vi "TR_KeyboardStatus.vi"(11 "Mouse in":refnum<class "Keyboard.lvclass">) -> ()   [LabVIEW 2021, in "InputDevice.lvlib" / "Keyboard.lvclass"]
uses:
  Keyboard.lvclass
  8ae88d8c-86e8-4183-9e02-5cb064982b42.vi
  <vilib>/Utility/inputDevices.llb/keyboardAcquire.vi
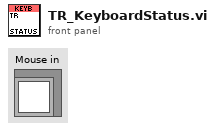
[diagram p1: front panel]
types:
  T1 = typedef "Keyboard.lvclass/data.ctl" = cluster{"DeviceID":refnum<k1>, "Key Pressed":refnum<user-event>, "KeyPressedEvents":refnum<event-registration>, "StopNotifier":refnum<notifier>}
  T2 = enum16{"0", "1", "2", "3", "4", "5", "6", "7", "8", "9", "A", "B", "C", "D", "E", "F", "G", "H", "I", "J", "K", "L", "M", "N", "O", "P", "Q", "R", "S", "T", "U", "V", "W", "X", "Y", "Z", "F1", "F2", "F3", "F4", "F5", "F6", "F7", "F8", "F9", "F10", "F11", "F12", "F13", "F14", "F15", "ADD", "BACK", "BACKSLASH", "CAPITAL", "COMMA", "DECIMAL", "DELETE", "DIVIDE", "DOWN", "END", "EQUALS", "ESCAPE", "GRAVE (`)", "HOME", "INSERT", "LBRACKET", "LCONTROL", "LEFT", "L ALT", "LSHIFT", "LWIN", "MINUS", "MULTIPLY", "NEXT", "NUMLOCK", "NUMPAD_0", "NUMPAD_1", "NUMPAD_2", "NUMPAD_3", "NUMPAD_4", "NUMPAD_5", "NUMPAD_6", "NUMPAD_7", "NUMPAD_8", "NUMPAD_9", "PAUSE", "PERIOD", "PRIOR (PG UP)", "RBRACKET", "RCONTROL", "RETURN", "RIGHT", "R ALT", "RSHIFT", "RWIN", "SCROLL", "SEMICOLON", "SLASH", "SPACE", "SUBTRACT", "TAB", "UP", "ENTER (num pad)", "' (quote)"}[]
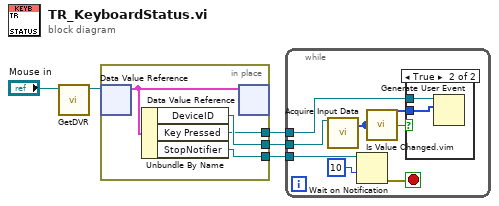
[diagram p0: block diagram]
diagram:
  n1 = call "GetDVR.vi"("Mouse"="Mouse in") -> ("DVR"=w4:refnum<data-value>)  [unwired: 9 in, 1 out]
  n2 = in-place {
    in-place-border: [w9] -> w3
    in-place-border: [w8] -> w2
    in-place-border: [w7] -> w1
    n3 = in-place-dvr #1(w4) -> (w6:T1)  [unwired: 1 out]
    n4 = Unbundle By Name(w6) -> ("DeviceID"=w9:refnum<k1>, "Key Pressed"=w8:refnum<user-event>, "StopNotifier"=w7:refnum<notifier>)
    n5 = in-place-dvr #1(w6) -> ()  [unwired: 2 out]
  }
  n6 = while {
    tunnel: w3 -> [w16]
    tunnel: w2 -> [w14]
    tunnel: w1 -> [w11]
    stop <- w12 stop-if-true
    n7 = call-poly <vilib>:"Acquire Input Data.vi"("device ID"=w16) -> ("keys pressed"=w13:T2)  [unwired: 16 in, 2 out]
    n8 = Wait on Notification(notifier=w11, timeout in ms (-1)=10) -> (error out=w12:errorcluster)  [unwired: 2 in, 3 out]
    n9 = call "Is Value Changed.vim"("value"=w13) -> ("changed or first call?"=w15:bool)
    n10 = case shown="True" w15 {
      tunnel: w14 -> [_ w18]
      tunnel: w13 -> [_ w17]
      frame False {
      }
      frame True {
        n11 = Generate User Event(user event=w18, event data cluster=w17) -> ()  [unwired: 2 in, 2 out]
      }
    }
  }
